vi "Kalman_Filter_Sub.vi"(6 "F  Matrix":T1, 7 "H Matrix":T1, 9 "Gyro":dbl format="%#_13g", 10 "Steady State Kalman Predictor Gain matrix":T1, 11 "accelerometer angle":dbl format="%#_13g") -> (3 "State Predicted Estimate X^(k+1/k)":dbl[](array[numeric]))   [LabVIEW 2020]
uses:
  <vilib>/Analysis/Matrix/Datatypes/RealMatrix.ctl
  <vilib>/Analysis/Matrix/NI_Matrix.lvlib
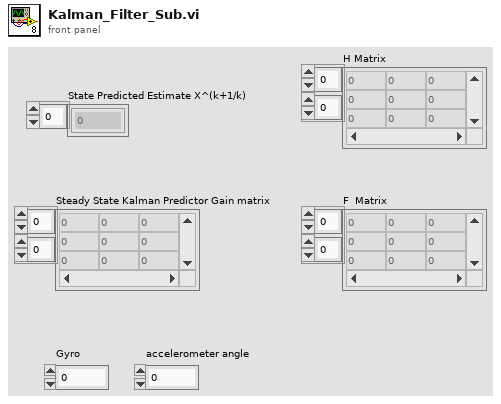
[diagram p1: front panel]
types:
  T1 = typedef "NI_Matrix.lvlib/RealMatrix.ctl" = dbl[][]
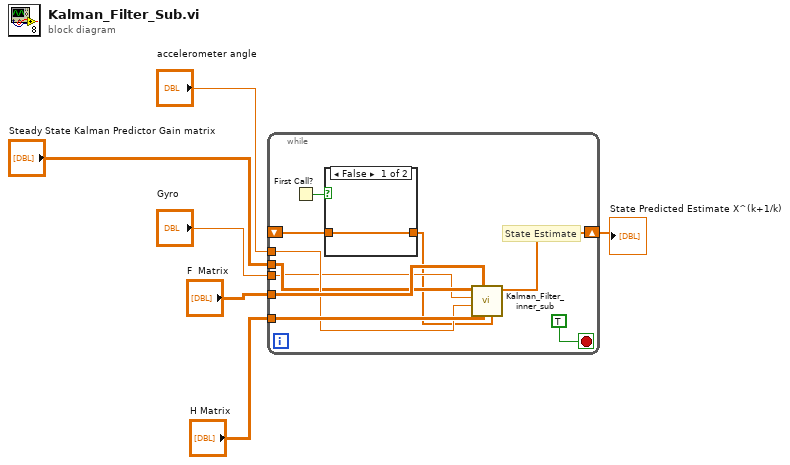
[diagram p0: block diagram]
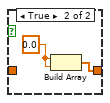
[diagram p2: hidden frame]
diagram:
  n1 = while {
    tunnel: "Steady State Kalman Predictor Gain matrix" -> [w9]
    tunnel: "F  Matrix" -> [w12]
    tunnel: "H Matrix" -> [w11]
    shift-right: [w13] -> w4
    shift-left: _ -> [w14]
    tunnel: "accelerometer angle" -> [w10]
    tunnel: "Gyro" -> [w8]
    stop <- TRUE stop-if-true
    # "State Estimate"
    n2 = First Call?() -> (First Call?: T/F=w15:bool)
    n3 = case shown="False" w15 {
      tunnel: w14 -> [w17 _]
      tunnel: [w17 w18] -> w7
      frame False {
      }
      frame True {
        w19 = 0.0 ("element")
        n4 = Build Array(w19, w19) -> (w18:dbl[])
      }
    }
    n5 = call "Kalman_Filter_inner_sub.vi"("X from register"=w7, "H Matrix"=w11, "F  Matrix"=w12, "Accelerometer ANGLE in degrees"=w10, "Gyro Velocity"=w8, "Steady State Kalman Predictor Gain matrix"=w9) -> ("X^ to register"=w13:dbl[])  [unwired: 5 in]
  }
  "State Predicted Estimate X^(k+1/k)" <- w4
